vi "Report Invalid DVR.vi"(8 "Error In":errorcluster, 11 "Invalid DVR":bool) -> (0 "Error Out":errorcluster)   [LabVIEW 2021, in "Utilities.lvlib"]
uses:
  Utilities.lvlib
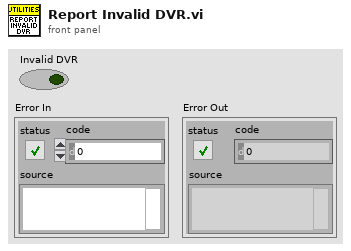
[diagram p1: front panel]
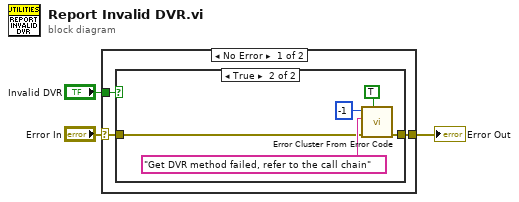
[diagram p0: block diagram]
diagram:
  n1 = case shown="No Error" "Error In" {
    selector: "Error In" -> [w6 w13]
    tunnel: [w5 w13] -> w2
    tunnel: "Invalid DVR" -> [w4 _]
    frame No Error {
      n2 = case shown="True" w4 {
        tunnel: [w7 w9] -> w5
        tunnel: w6 -> [w7 w8]
        frame False {
        }
        frame True {
          n3 = call <vilib>:"Error Cluster From Error Code.vi"("show call chain? (False)"=TRUE, "error in (no error)"=w8, "error message (\"\")"="Get DVR method failed, refer to the call chain" ("error message (\"\")"), "error code (0)"=-1) -> ("error out"=w9:errorcluster)  [unwired: 5 in]
        }
      }
    }
    frame Error {
    }
  }
  "Error Out" <- w2
